vi "Averaging.vi"(0 "VISA IN":refnum<visa-resource-name>, 2 "AVG":i32, 3 "Average ON/OFF":bool, 5 "error in":errorcluster, 6 "Channel":i32=1) -> (14 "VISA Out":refnum<visa-resource-name>, 19 "error out":errorcluster)   [LabVIEW 2018, in "PNA-X.lvlib"]
uses:
  PNA-X.lvlib
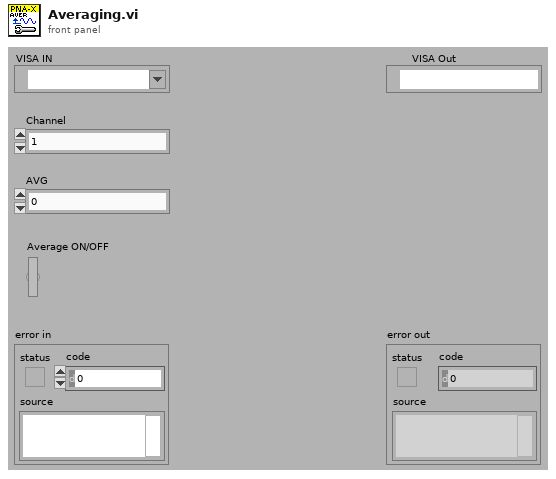
[diagram p1: front panel]
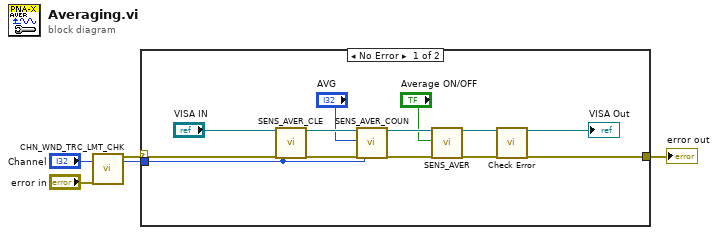
[diagram p0: block diagram]
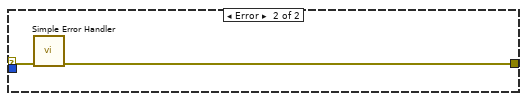
[diagram p2: hidden frame]
diagram:
  n1 = call "CHN_WND_TRC_LMT_CHK.vi"("Channel"="Channel", "error in"="error in") -> ("error out"=w2:errorcluster, "Channel"=w1:i32)  [unwired: 13 in, 3 out]
  n2 = case shown="No Error" w2 {
    selector: w2 -> [w9 w20]
    tunnel: [w17 w19] -> w4
    tunnel: w1 -> [w8 _]
    frame No Error {
      n3 = call "SENS_AVER_CLE.vi"("VISA IN"="VISA IN", "error in"=w9, "Channel"=w8) -> ("VISA Out"=w15:refnum<visa-resource-name>, "error out"=w10:errorcluster)  [unwired: 15 in]
      n4 = call "SENS_AVER_COUN.vi"("VISA IN"=w15, "AVG"="AVG", "error in"=w10, "Channel"=w8) -> ("VISA Out"=w14:refnum<visa-resource-name>, "error out"=w11:errorcluster)  [unwired: 14 in]
      n5 = call "SENS_AVER.vi"("VISA IN"=w14, "Average ON/OFF"="Average ON/OFF", "error in"=w11) -> ("VISA Out"=w13:refnum<visa-resource-name>, "error out"=w12:errorcluster)  [unwired: 15 in]
      n6 = call "Check Error.vi"("VISA Resource Name"=w13, "error in (no error)"=w12) -> ("dup VISA session"=→"VISA Out":refnum<visa-resource-name>, "error out"=w17:errorcluster)  [unwired: 16 in]
    }
    frame Error {
      n7 = call <vilib>:"Simple Error Handler.vi"("error in (no error)"=w20) -> ("error out"=w19:errorcluster)  [unwired: 4 in, 4 out]
    }
  }
  "error out" <- w4
